vi "4.vi"() -> ()   [LabVIEW 2018]
panel:
  out "x > 0?":bool
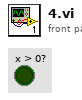
[diagram p1: front panel]
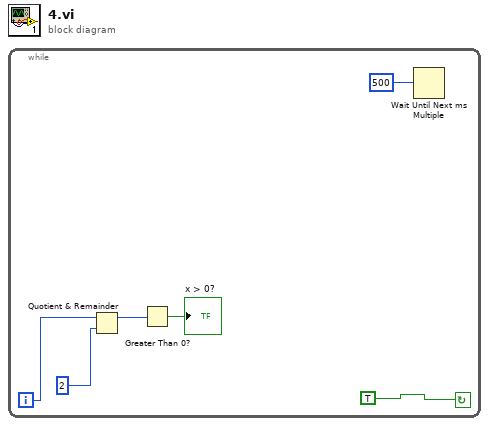
[diagram p0: block diagram]
diagram:
  n1 = while {
    i -> [w4]
    stop <- TRUE continue-if-true
    n2 = Quotient & Remainder(x=w4, y=2) -> (x-y*floor(x/y)=w3:i32)  [unwired: 1 out]
    n3 = Greater Than 0?(x=w3) -> (x > 0?=→"x > 0?":bool)
    n4 = Wait Until Next ms Multiple(millisecond multiple=500) -> ()  [unwired: 1 out]
  }
